vi "Re-establish Device on Microgrid.vi"(7 "Activate":bool=TRUE, 8 "error in":errorcluster, 9 "Mode":T1, 10 "DeviceID":T2, 11 "Generic Optimization in":refnum<class "Generic Optimization.lvclass">) -> (0 "error out":errorcluster, 3 "Generic Optimization out":refnum<class "Generic Optimization.lvclass">)   [LabVIEW 2018, in "Generic Optimization Actor.lvlib" / "Generic Optimization.lvclass"]
uses:
  Generic Optimization.lvclass
  C:/Users/Administrator/Desktop/2018LabVIEW EMS/EMS Generic Actor/EMS Generic/EMS Generic.lvclass
  C:/Program Files (x86)/National Instruments/LabVIEW 2018/vi.lib/ActorFramework/Actor/Actor.lvclass
  C:/Users/Administrator/Desktop/2018LabVIEW EMS/Device Communication and Control Abstract Actor/Device Communication and Control Abstract/Device Communication and Control Abstract.lvclass
  <vilib>/ORNL/CSEISMIC DDS/CSEISMIC DDS Base/Data Types/Controls/DeviceID.ctl
  <vilib>/ORNL/CSEISMIC DDS/CSEISMIC DDS Base/Data Types/Controls/Generation Mode.ctl
  <vilib>/ORNL/CSEISMIC DDS/CSEISMIC DDS Base/Data Types/IED_setMicrogridID.ctl
  EMS Core/EMS Messages/IED setMicrogridID (Single) Msg/IED setMicrogridID (Single) Msg.lvclass
  C:/Users/Administrator/Desktop/2018LabVIEW EMS/Device Communication and Control Abstract Actor/Device Communication and Control Abstract Messages/Set Single Device IED MicrogridID Msg/Set Single Device IED MicrogridID Msg.lvclass
  <vilib>/ORNL/CSEISMIC DDS/CSEISMIC DDS Base/Data Types/DER_setGenerationMode.ctl
  <vilib>/ActorFramework/Actor/Actor.lvclass/Actor.ctl
  Device Communication and Control Abstract Actor/Device Communication and Control Abstract Messages/Set Single Device IED MicrogridID Msg/Set Single Device IED MicrogridID Msg.lvclass/Set Single Device IED MicrogridID Msg.ctl
  <vilib>/ActorFramework/Message Enqueuer/Message Enqueuer.lvclass/Message Enqueuer.ctl
  Device Communication and Control Abstract Actor/Device Communication and Control Abstract/Device Communication and Control Abstract.lvclass/Device Communication and Control Abstract.ctl
  Device Communication and Control Abstract Actor/Device Communication and Control Abstract Messages/Set DER GenerationMode Msg/Set DER GenerationMode Msg.lvclass/Set DER GenerationMode Msg.ctl
  <vilib>/ORNL/CSEISMIC DDS/CSEISMIC DDS Base/Data Types/DER_Control.ctl
  Device Communication and Control Abstract Actor/Device Communication and Control Abstract Messages/Set DER Control Msg/Set DER Control Msg.lvclass/Set DER Control Msg.ctl
  <vilib>/ActorFramework/Message Enqueuer/Enqueue.vi
  Device Communication and Control Abstract Actor/Device Communication and Control Abstract Messages/Set DER GenerationMode Msg/Send Delayed Set DER GenerationMode.vi
  Device Communication and Control Abstract Actor/Device Communication and Control Abstract Messages/Set DER Control Msg/Send Delayed Set DER Control.vi
  Device Communication and Control Abstract Actor/Device Communication and Control Abstract Messages/Set Single Device IED MicrogridID Msg/Set Single Device IED MicrogridID Msg.lvclass
  C:/Program Files (x86)/National Instruments/LabVIEW 2018/vi.lib/ActorFramework/Message/Message.lvclass
  Device Communication and Control Abstract Actor/Device Communication and Control Abstract/Device Communication and Control Abstract.lvclass
  Device Communication and Control Abstract Actor/Device Communication and Control Abstract Messages/Set DER GenerationMode Msg/Set DER GenerationMode Msg.lvclass
  Device Communication and Control Abstract Actor/Device Communication and Control Abstract Messages/Set DER Control Msg/Set DER Control Msg.lvclass
  <vilib>/ActorFramework/Message Priority Queue/Priority Enqueue.vi
  <vilib>/ActorFramework/Time-Delayed Send Message/Time-Delayed Send Message.vi
  <vilib>/ActorFramework/Actor/Actor.lvclass
  <vilib>/ORNL/CSEISMIC DDS/CSEISMIC DDS Base/CSEISMIC DDS.lvclass
  EMS Generic Actor/EMS Generic/EMS Generic.lvclass
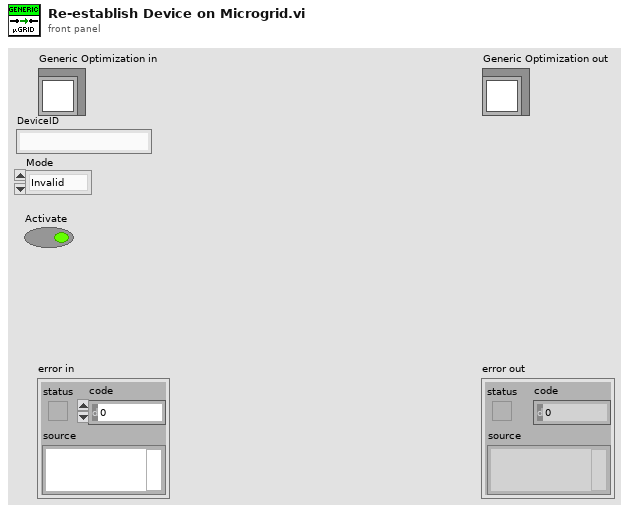
[diagram p1: front panel]
types:
  T1 = typedef "CSEISMIC DDS.lvlib/CSEISMIC DDS.lvclass/Generation Mode.ctl" = enum32{"Invalid", "PQ", "Droop", "PV", "PF", "VF"}
  T2 = typedef "CSEISMIC DDS.lvlib/CSEISMIC DDS.lvclass/DeviceID.ctl" = string
  T3 = typedef "CSEISMIC DDS.lvlib/CSEISMIC DDS.lvclass/DER_setGenerationMode.ctl" = cluster{"DeviceID":T2, "Mode":T1}
  T4 = typedef "CSEISMIC DDS.lvlib/CSEISMIC DDS.lvclass/IED_setMicrogridID.ctl" = cluster{"DeviceID":T2, "MicrogridID":u8}
  T5 = typedef "CSEISMIC DDS.lvlib/CSEISMIC DDS.lvclass/DER_Control.ctl" = cluster{"DeviceID":T2, "Activate":bool, "Deactivate":bool}
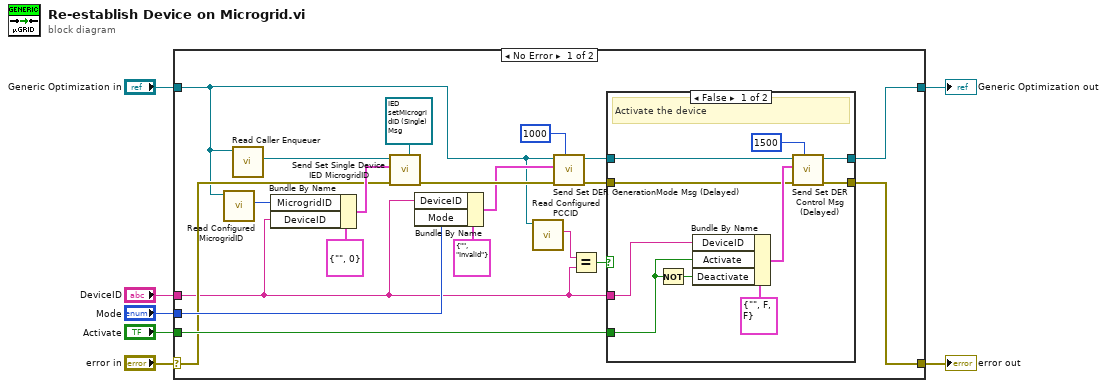
[diagram p0: block diagram]
diagram:
  n1 = case shown="No Error" "error in" {
    selector: "error in" -> [w19 w41]
    tunnel: [w18 w41] -> w6
    tunnel: [w17 w40] -> w4
    tunnel: "Generic Optimization in" -> [w11 w40]
    tunnel: "DeviceID" -> [w9 _]
    tunnel: "Mode" -> [w21 _]
    tunnel: "Activate" -> [w20 _]
    frame No Error {
      n2 = call "Read Configured MicrogridID.vi"("EMS Generic in"=w11) -> ("Microgrid ID"=w25:u8)  [unwired: 8 in, 2 out]
      n3 = call <vilib>:"Read Caller Enqueuer.vi"("Actor"=w11) -> ("Caller Enqueuer"=w27:refnum<class "Message Enqueuer.lvclass">)  [unwired: 10 in]
      n4 = Bundle By Name(cluster=T4 {"DeviceID"="", "MicrogridID"=0} ("IED_setMicrogridID"), "MicrogridID"=w25, "DeviceID"=w9) -> (w24:T4)
      n5 = call "Send Set Single Device IED MicrogridID.vi"("Message Type"=refnum<class "IED setMicrogridID (Single) Msg.lvclass"> refnum ("SCADA Core.lvlib:IED setMicrogridID (Single) Msg.lvclass"), "error in (no error)"=w19, "IED_setMicrogridID"=w24, "Message Enqueuer"=w27) -> ("error out"=w16:errorcluster)  [unwired: 6 in, 1 out]
      n6 = Bundle By Name(cluster=T3 {"DeviceID"="", "Mode"=enum."Invalid"} ("DER_setGenerationMode"), "DeviceID"=w9, "Mode"=w21) -> (w13:T3)
      n7 = call "Read Configured PCCID.vi"("EMS Generic in"=w11) -> ("PCCID"=w10:T2)  [unwired: 8 in, 2 out]
      n8 = call "Send Set DER GenerationMode Msg (Delayed).vi"("Milliseconds To Wait (1000)"=1000 ("Milliseconds To Wait"), "error in"=w16, "DER_setGenerationMode"=w13, "SCADA Sub Abstract in"=w11) -> ("error out"=w15:errorcluster, "dup SCADA Sub Abstract"=w14:refnum<class "Generic Optimization.lvclass">)  [unwired: 6 in]
      n9 = Equal?(x=w10, y=w9) -> (x = y?=w8:bool)
      n10 = case shown="False" w8 {
        tunnel: w20 -> [w36 _]
        tunnel: w9 -> [w34 _]
        tunnel: [w33 w38] -> w18
        tunnel: [w31 w39] -> w17
        tunnel: w15 -> [w29 w38]
        tunnel: w14 -> [w28 w39]
        frame False {
          # "Activate the device"
          n11 = Not(x=w36) -> (.not. x?=w35:bool)
          n12 = Bundle By Name(cluster=T5 {"DeviceID"="", "Activate"=FALSE, "Deactivate"=FALSE} ("DER_Control"), "DeviceID"=w34, "Activate"=w36, "Deactivate"=w35) -> (w32:T5)
          n13 = call "Send Set DER Control Msg (Delayed).vi"("Milliseconds To Wait (1000)"=1500 ("Milliseconds To Wait"), "error in"=w29, "DER_Control"=w32, "SCADA Sub Abstract in"=w28) -> ("error out"=w33:errorcluster, "dup SCADA Sub Abstract"=w31:refnum<class "Generic Optimization.lvclass">)  [unwired: 6 in]
        }
        frame True {
          # "We don't want to automatically send Activate (resync) to the PCC"
        }
      }
    }
    frame Error {
    }
  }
  "error out" <- w6
  "Generic Optimization out" <- w4
